vi "Fetch From Buffer (Multiple Points).vi"(6 "Buffer Elements":u16(ring)=7 items=["Date", "Extra", "Formatted", "Fractional", "Relative", "Seconds", "Status", "Time", "Timestamp", "Unit"], 8 "error in (no error)":errorcluster, 9 "Timeout (10000 ms)":i32=10000 format="%#.6g", 10 "Buffer Name":string="defbuffer2", 11 "VISA resource name":refnum<visa-resource-name>="DMM1") -> (0 "error out":errorcluster={"status"=TRUE, "code"=-1073807194, "source"="Keithley DMM7510.lvlib:Get Buffer Actual Readings Count.vi->Keithley DMM7510.lvlib:Fetch From Buffer (Multiple Points).vi中的VISA写入"}, 1 "Element Value":string[](array[string]), 3 "VISA resource name out":refnum<visa-resource-name>="DMM1")   [LabVIEW 2015, in "Keithley DMM7510.lvlib"]
doc: "Reads and returns multiple measurements from the instrument. Returns specified data elements from a specified reading buffer. This VI does not initiate a trigger."
uses:
  Keithley DMM7510.lvlib
  <vilib>/Analysis/baseanly.llb/Mean (DBL).vi
  <vilib>/Analysis/NI_AALBase.lvlib
panel:
  out "大小":i32
  out "mean":dbl=nan caption="均值" format="%0.2f"
  out "波形图":dbl[](graph)
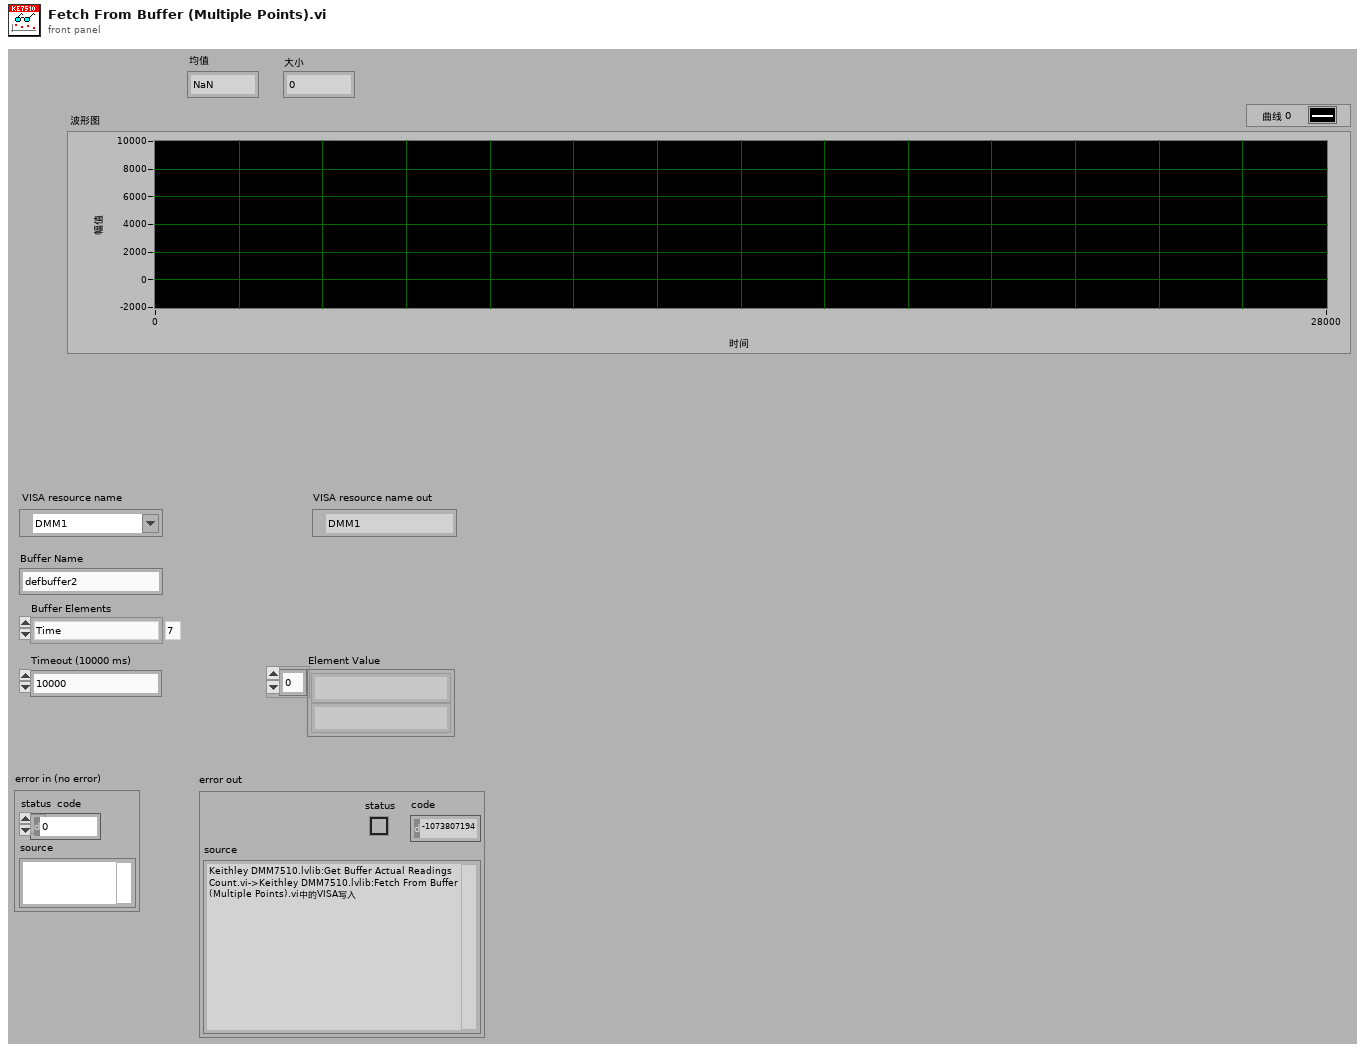
[diagram p1: front panel]
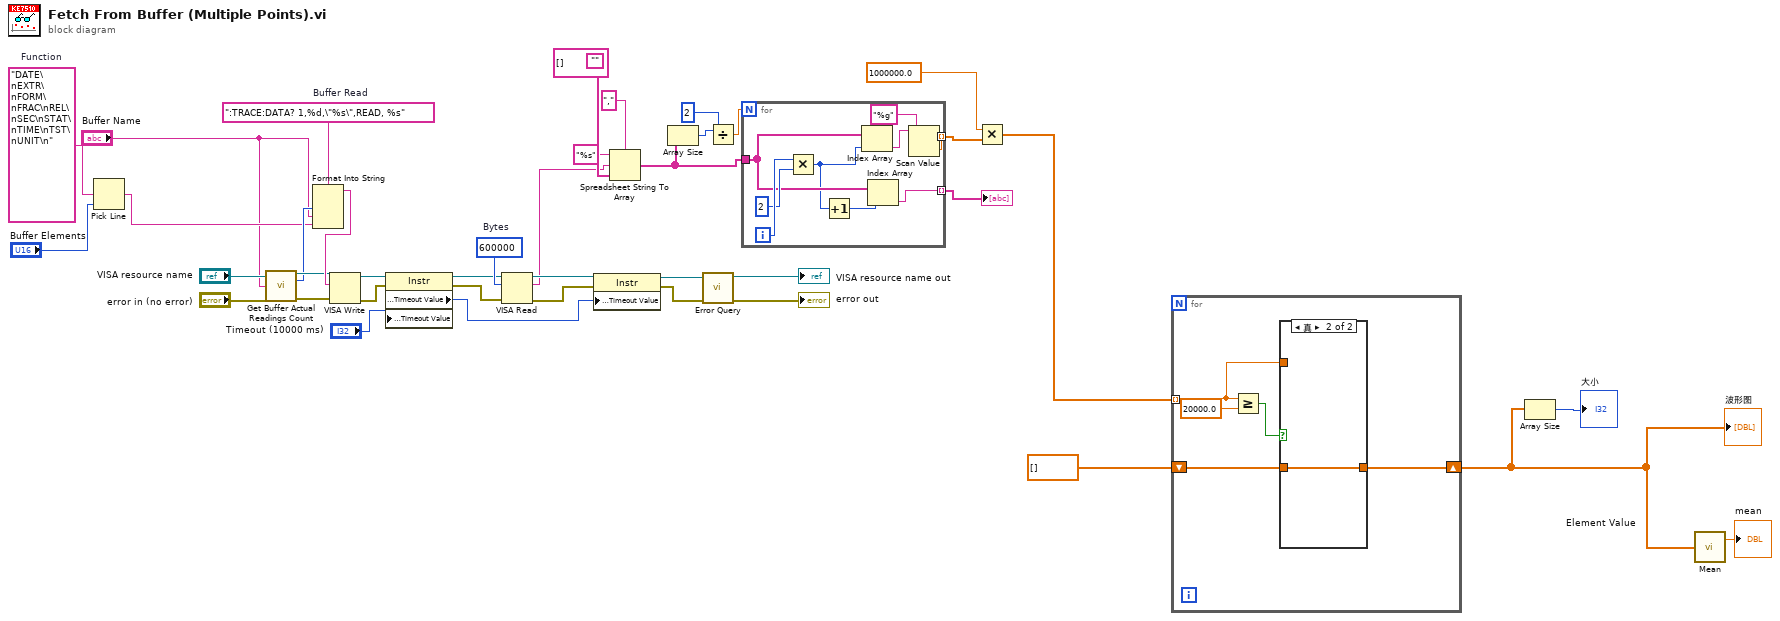
[diagram p0: block diagram]
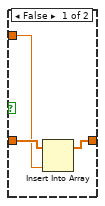
[diagram p2: hidden frame]
diagram:
  (unwired) ""
  w24 = "DATE\nEXTR\nFORM\nFRAC\nREL\nSEC\nSTAT\nTIME\nTST\nUNIT\n"  # Function
  w27 = ":TRACE:DATA? 1,%d,\"%s\",READ, %s"  # Buffer Read
  w40 = u32 600000  # Bytes
  n1 = Pick Line(multi-line string=w24, line index="Buffer Elements") -> (output string=w9:string)  [unwired: 1 out]
  n2 = call "Get Buffer Actual Readings Count.vi"("VISA resource name"="VISA resource name", "Buffer Name (defbuffer1)"="Buffer Name", "error in (no error)"="error in (no error)") -> ("VISA resource name out"=w11:refnum<visa-resource-name>, "Actual Readings"=w10:i32, "error out"=w12:errorcluster)  [unwired: 10 in]
  n3 = Format Into String(format string=w27, w10, "Buffer Name", w9) -> (resulting string=w26:string)  [unwired: 2 in, 1 out]
  n4 = VISA Write(VISA resource name=w11, write buffer=w26, error in (no error)=w12) -> (VISA resource name out=w37:refnum<visa-resource-name>, error out=w36:errorcluster)  [unwired: 1 out]
  n5 = property class="Instr"(reference=w37, error in=w36, "General Settings:Timeout Value"="Timeout (10000 ms)") -> (reference out=w35:refnum<visa-resource-name>, error out=w34:errorcluster, "General Settings:Timeout Value"=w28:u32)
  n6 = VISA Read(VISA resource name=w35, byte count=w40, error in (no error)=w34) -> (VISA resource name out=w32:refnum<visa-resource-name>, read buffer=w15:string, error out=w30:errorcluster)  [unwired: 1 out]
  n7 = property class="Instr"(reference=w32, error in=w30, "General Settings:Timeout Value"=w28) -> (reference out=w31:refnum<visa-resource-name>, error out=w29:errorcluster)
  n8 = Spreadsheet String To Array(delimiter (Tab)=",", format string="%s", spreadsheet string=w15, array type (2D Dbl)=string[] []) -> (array=w21:string[])
  n9 = Array Size(array=w21) -> (size(s)=w19:i32)
  n10 = call "Error Query.vi"("error in (no error)"=w29, "VISA resource name"=w31) -> ("error out"=→"error out":errorcluster, "VISA resource name out"=→"VISA resource name out":refnum<visa-resource-name>)  [unwired: 6 in, 2 out]
  n11 = Divide(x=w19, y=2) -> (x/y=w17:dbl)
  n12 = for {
    N: w17 -> [_]
    tunnel: w21 -> [w47]
    tunnel: [w42] -> w7 mode=indexing
    tunnel: [w45] -> w16 mode=indexing
    i -> [w49]
    n13 = Multiply(x=w49, y=2) -> (x*y=w41:i32)
    n14 = Increment(x=w41) -> (x+1=w46:i32)
    n15 = Index Array(array=w47, index=w41) -> (element=w44:string)
    n16 = Index Array(array=w47, index=w46) -> (element=w45:string)
    n17 = Scan Value(string=w44, format string="%g") -> (value=w42:dbl)  [unwired: 1 in, 1 out]
  }
  "Element Value" <- w16
  n18 = Multiply(x=1000000.0, y=w7) -> (x*y=w4:dbl[])
  n19 = for {
    tunnel: w4 -> [w52] mode=indexing
    shift-right: [w50] -> w2
    shift-left: dbl[] [] -> [w53]
    n20 = Greater Or Equal?(x=w52, y=20000.0) -> (x >= y?=w51:bool)
    n21 = case shown="真" w51 {
      tunnel: w53 -> [w57 w58]
      tunnel: w52 -> [w56 _]
      tunnel: [w55 w58] -> w50
      frame False {
        n22 = Insert Into Array(array=w57, new element=w56) -> (w55:dbl[])  [unwired: 1 in]
      }
      frame True {
      }
    }
  }
  "波形图" <- w2
  n23 = Array Size(array=w2) -> (size(s)=→"大小":i32)
  n24 = call-poly <vilib>:"Mean.vi"("X"=w2) -> ("mean"=→"mean":dbl)  [unwired: 1 out]
